vi "Mysql data reader 2D string.vi"(8 "error in (no error)":errorcluster, 11 ".NET Refnum in":refnum<k24>) -> (0 "error out":errorcluster, 3 "Array":string[][](array[string]))   [LabVIEW 2020, in "mysql.lvlib" / "mysql.lvclass"]
uses:
  mysql.lvclass
  MySql.Data
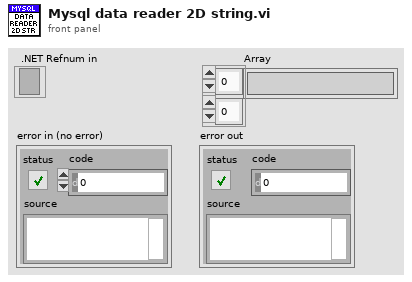
[diagram p1: front panel]
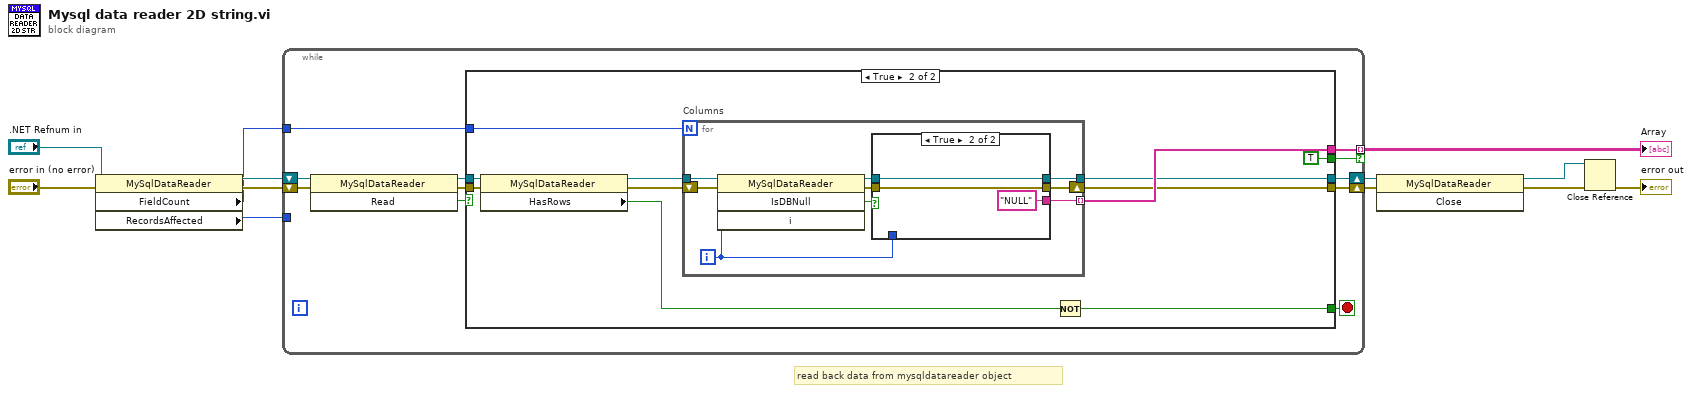
[diagram p0: block diagram]
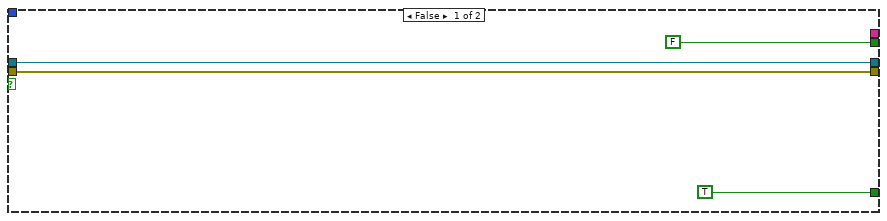
[diagram p2: hidden frame]
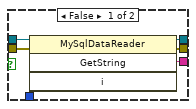
[diagram p3: hidden frame]
diagram:
  # "read back data from mysqldatareader object"
  n1 = property class="MySqlDataReader"(reference=".NET Refnum in", error in="error in (no error)") -> (reference out=w7:refnum<k24>, error out=w6:errorcluster, "FieldCount"=w3:i32, "RecordsAffected"=w12:i32)
  n2 = while {
    tunnel: w3 -> [w23]
    tunnel: [w22] -> w4 mode=indexing if=w13
    shift-right: [w16] -> w9
    shift-left: w6 -> [w21]
    shift-right: [w17] -> w8
    shift-left: w7 -> [w19]
    tunnel: w12 -> [_]
    stop <- w15 stop-if-true
    n3 = invoke class="MySqlDataReader" method="Read"(reference=w19, error in=w21) -> (reference out=w18:refnum<k24>, error out=w20:errorcluster, "Read"=w14:bool)  [unwired: 1 in]
    n4 = case shown="True" w14 {
      tunnel: w23 -> [_ w38]
      tunnel: [_ w37] -> w22
      tunnel: w20 -> [w25 w36]
      tunnel: w18 -> [w26 w35]
      tunnel: [w26 w34] -> w17
      tunnel: [w25 w30] -> w16
      tunnel: [TRUE ("HasRows") w28] -> w15
      tunnel: [FALSE TRUE] -> w13
      frame False {
      }
      frame True {
        n5 = property class="MySqlDataReader"(reference=w35, error in=w36) -> (reference out=w33:refnum<k24>, error out=w32:errorcluster, "HasRows"=w31:bool)
        n6 = for "Columns" {
          N: w38 -> [_]
          tunnel: w33 -> [w42]
          shift-right: [w47] -> w30
          shift-left: w32 -> [w43]
          tunnel: [w46] -> w37 mode=indexing
          tunnel: [w45] -> w34
          i -> [w44]
          n7 = invoke class="MySqlDataReader" method="IsDBNull"(reference=w42, error in=w43, "i"=w44) -> (reference out=w41:refnum<k24>, error out=w40:errorcluster, "IsDBNull"=w39:bool)  [unwired: 1 in, 1 out]
          n8 = case shown="True" w39 {
            tunnel: [w53 w55] -> w47
            tunnel: [w52 "NULL" ("GetString")] -> w46
            tunnel: [w51 w56] -> w45
            tunnel: w44 -> [w50 _]
            tunnel: w41 -> [w49 w56]
            tunnel: w40 -> [w48 w55]
            frame False {
              n9 = invoke class="MySqlDataReader" method="GetString"(reference=w49, error in=w48, "i"=w50) -> (reference out=w51:refnum<k24>, error out=w53:errorcluster, "GetString"=w52:string)  [unwired: 1 in, 1 out]
            }
            frame True {
            }
          }
        }
        n10 = Not(x=w31) -> (.not. x?=w28:bool)
      }
    }
  }
  "Array" <- w4
  n11 = invoke class="MySqlDataReader" method="Close"(reference=w8, error in=w9) -> (reference out=w11:refnum<k24>, error out=w10:errorcluster)  [unwired: 1 in, 1 out]
  n12 = Close Reference(reference=w11, error in (no error)=w10) -> (error out=→"error out":errorcluster)
